vi "AlliGator Find Closest Valid Calibration Phasor.vi"(9 "Dataset Series Index":i32, 10 "phi Array":dbl[](array[numeric]), 11 "m Array":dbl[](array[numeric])) -> (1 "Found?":bool, 2 "phi":dbl, 3 "m":dbl)   [LabVIEW 2021, in "AlliGator Phasor Calibration.lvlib"]
doc: "Going backwards and forwards in the calibration series, starting from the <B>Dataset Series Index</B>, finds the first valid calibration phasor and returns it.\n\nIf none is found (bogus series), setd the <B>Found></B> flag to false."
uses:
  AlliGator Phasor Calibration.lvlib
panel:
  # "see the AlliGator License on the block diagram (Ctrl+E or Window:Show Block Diagram)"
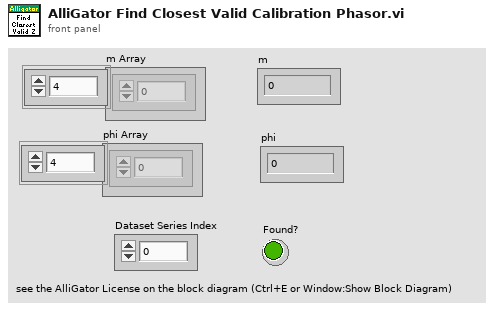
[diagram p1: front panel]
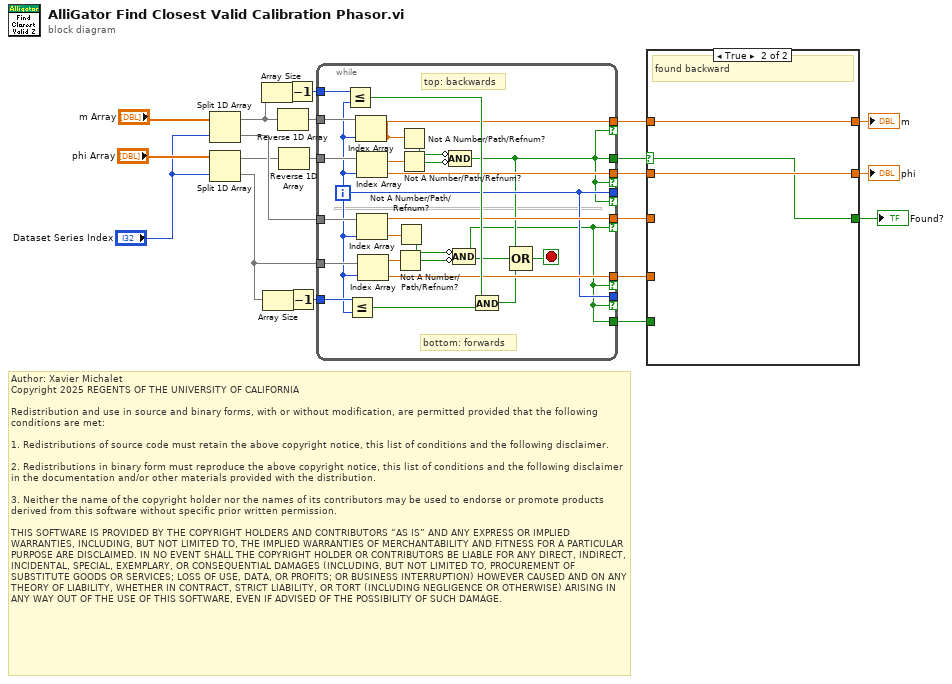
[diagram p0: block diagram]
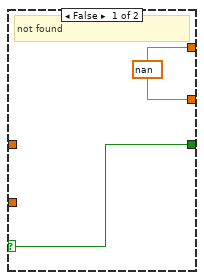
[diagram p3: hidden frame]
diagram:
  # "Author: Xavier Michalet\nCopyright 2025 REGENTS OF THE UNIVERSITY OF CALIFORNIA\n\nRedistribution and use in source and binary forms, with or without modification, are permitted provided that the following conditions are met:\n\n1. Redistributions of source code must retain the above copyright notice, this list of conditions and the following disclaimer.\n\n2. Redistributions in binary form must reproduce the above copyright notice, this list of conditions and the following disclaimer in the documentation and/or other materials provided with the distribution.\n\n3. Neither the name of the copyright holder nor the names of its contributors may be used to endorse or promote products derived from this software without specific prior written permission.\n\nTHIS SOFTWARE IS PROVIDED BY THE COPYRIGHT HOLDERS AND CONTRIBUTORS “AS IS” AND ANY EXPRESS OR IMPLIED WARRANTIES, INCLUDING, BUT NOT LIMITED TO, THE IMPLIED WARRANTIES OF MERCHANTABILITY AND FITNESS FOR A PARTICULAR PURPOSE ARE DISCLAIMED. IN NO EVENT SHALL THE COPYRIGHT HOLDER OR CONTRIBUTORS BE LIABLE FOR ANY DIRECT, INDIRECT, INCIDENTAL, SPECIAL, EXEMPLARY, OR CONSEQUENTIAL DAMAGES (INCLUDING, BUT NOT LIMITED TO, PROCUREMENT OF SUBSTITUTE GOODS OR SERVICES; LOSS OF USE, DATA, OR PROFITS; OR BUSINESS INTERRUPTION) HOWEVER CAUSED AND ON ANY THEORY OF LIABILITY, WHETHER IN CONTRACT, STRICT LIABILITY, OR TORT (INCLUDING NEGLIGENCE OR OTHERWISE) ARISING IN ANY WAY OUT OF THE USE OF THIS SOFTWARE, EVEN IF ADVISED OF THE POSSIBILITY OF SUCH DAMAGE."
  n1 = Split 1D Array(array="m Array", index="Dataset Series Index") -> (first subarray=w16:dbl[], second subarray=w20:dbl[])
  n2 = Split 1D Array(array="phi Array", index="Dataset Series Index") -> (first subarray=w19:dbl[], second subarray=w15:dbl[])
  n3 = Array Size(array=w16) -> (size(s)=w13:i32)
  n4 = Array Size(array=w15) -> (size(s)=w14:i32)
  n5 = Reverse 1D Array(array=w16) -> (reversed array=w18:dbl[])
  n6 = Reverse 1D Array(array=w19) -> (reversed array=w17:dbl[])
  n7 = Decrement(x=w13) -> (x-1=w12:i32)
  n8 = Decrement(x=w14) -> (x-1=w11:i32)
  n9 = while {
    tunnel: w18 -> [w43]
    tunnel: w20 -> [w41]
    tunnel: w17 -> [w42]
    tunnel: w15 -> [w40]
    tunnel: w11 -> [w34]
    tunnel: w12 -> [w35]
    tunnel: [w30] -> w4 if=w24
    tunnel: [w29] -> w3 if=w24
    tunnel: [w28] -> w7 if=w25
    tunnel: [w27] -> w9 if=w25
    tunnel: [w26] -> _ if=w25
    tunnel: [w26] -> _ if=w24
    tunnel: [w25] -> w10
    tunnel: [w24] -> w5
    i -> [w26]
    stop <- w31 stop-if-true
    # "bottom: forwards"
    # "top: backwards"
    n10 = Less Or Equal?(x=w35, y=w26) -> (x <= y?=w32:bool)
    n11 = Less Or Equal?(x=w34, y=w26) -> (x <= y?=w33:bool)
    n12 = Index Array(array=w43, index=w26) -> (element=w27:dbl)
    n13 = Index Array(array=w42, index=w26) -> (element=w28:dbl)
    n14 = Index Array(array=w41, index=w26) -> (element=w30:dbl)
    n15 = Index Array(array=w40, index=w26) -> (element=w29:dbl)
    n16 = Not A Number/Path/Refnum?(number/path/refnum=w29) -> (NaN/Path/Refnum?=w36:bool)
    n17 = Not A Number/Path/Refnum?(number/path/refnum=w30) -> (NaN/Path/Refnum?=w37:bool)
    n18 = Not A Number/Path/Refnum?(number/path/refnum=w27) -> (NaN/Path/Refnum?=w39:bool)
    n19 = Not A Number/Path/Refnum?(number/path/refnum=w28) -> (NaN/Path/Refnum?=w38:bool)
    n20 = Compound Arithmetic op=AND(invert w39, invert w38) -> (w25:bool)
    n21 = Compound Arithmetic op=AND(invert w37, invert w36) -> (w24:bool)
    n22 = And(x=w32, y=w33) -> (x .and. y?=w23:bool)
    n23 = Compound Arithmetic op=OR(w25, w24, w23) -> (w31:bool)
  }
  n24 = case shown="True" w10 {
    selector: w10 -> [_ w55]
    tunnel: w9 -> [_ w57]
    tunnel: [w47 w57] -> w8
    tunnel: w7 -> [_ w56]
    tunnel: [w46 w56] -> w6
    tunnel: w5 -> [w49 _]
    tunnel: w4 -> [w48 _]
    tunnel: w3 -> [w45 _]
    tunnel: [w44 w55] -> w1
    frame False {
      n25 = case shown="True" w49 {
        selector: w49 -> [w50 w52]
        tunnel: w48 -> [_ w54]
        tunnel: [w51 w54] -> w47
        tunnel: [w51 w53] -> w46
        tunnel: w45 -> [_ w53]
        tunnel: [w50 w52] -> w44
        frame False {
          w51 = nan ("Numeric Control")
          # "not found"
        }
        frame True {
          # "found forward"
        }
      }
    }
    frame True {
      # "found backward"
    }
  }
  "m" <- w8
  "phi" <- w6
  "Found?" <- w1
